vi "Create Protected Methods Folder.vi"   [LabVIEW 2015]
uses:
  Project Manipulation Scripts/Project Manipulation Scripts.lvlib
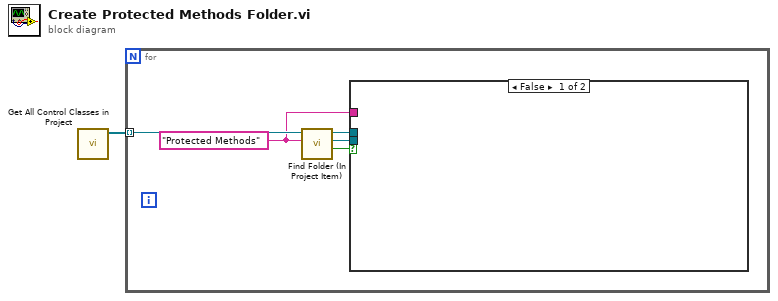
[diagram p0: block diagram]
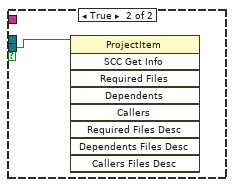
[diagram p2: hidden frame]
diagram:
  n1 = call "Get All Control Classes in Project.vi"() -> ("All Control Classes"=w1:refnum<vi>[])  [unwired: 11 in]
  n2 = for {
    tunnel: w1 -> [w6] mode=indexing
    w2 = "Protected Methods" ("Folder Name")
    n3 = call "Find Folder (In Project Item).vi"("Folder Name"=w2, "ProjectItem in"=w6) -> ("Found?"=w5:bool, "Folder Refnum"=w4:refnum<vi>, "ProjectItem out"=w3:refnum<vi>)  [unwired: 7 in]
    n4 = case shown="False" w5 {
      tunnel: w4 -> [_ w7]
      tunnel: w3 -> [_ _]
      tunnel: w2 -> [_ _]
      frame False {
      }
      frame True {
        n5 = invoke class="ProjectItem" method="SCC Get Info"(reference=w7) -> ()  [unwired: 8 in, 9 out]
      }
    }
  }
